vi "Storage Data.vi"(8 "Error In":errorcluster, 9 "Time Out In ms":i32=-1, 10 "Data In":variant, 11 "1D U16 Group With ID DVR Queue in":refnum<class "2D U16 Group With ID DVR Queue.lvclass">) -> (0 "Error Out":errorcluster, 1 "Time Out":bool, 3 "1D U16 Group With ID DVR Queue out":refnum<class "2D U16 Group With ID DVR Queue.lvclass">)   [LabVIEW 2024, in "2D U16 Group With ID DVR Queue.lvclass"]
uses:
  2D U16 Group With ID DVR Queue.lvclass
  Type Def/Data Type.ctl
  2D U16 Group With ID DVR Queue.lvclass/2D U16 Group With ID DVR Queue.ctl
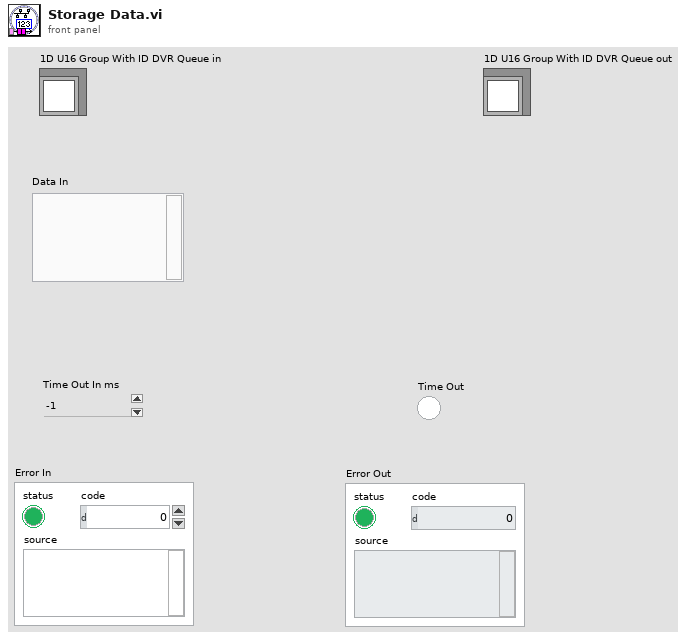
[diagram p1: front panel]
types:
  T1 = typedef "Data Type.ctl" = cluster{"Data ID":i64, "U16 Data Group":cluster{"Array":u16[][]}[]}
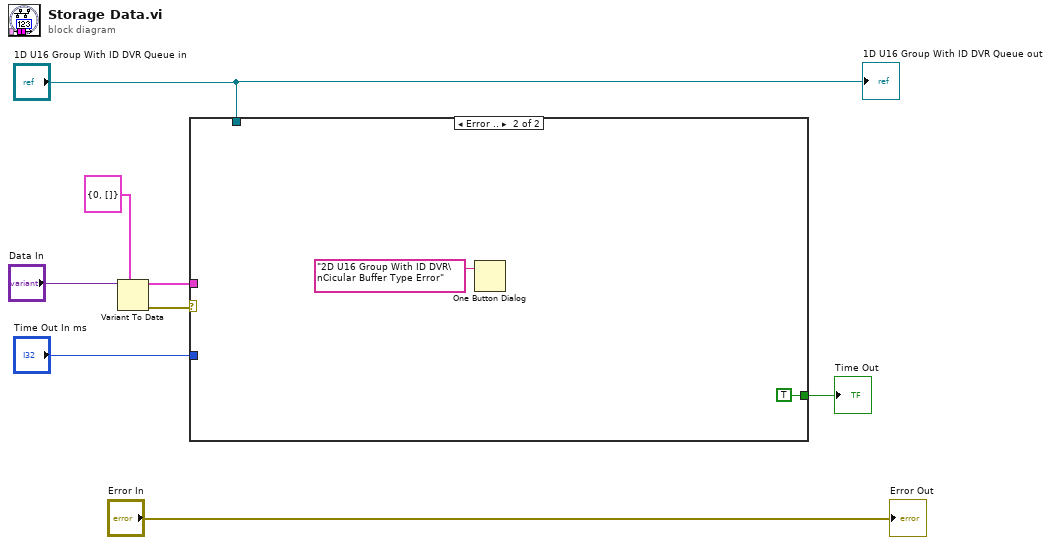
[diagram p0: block diagram]
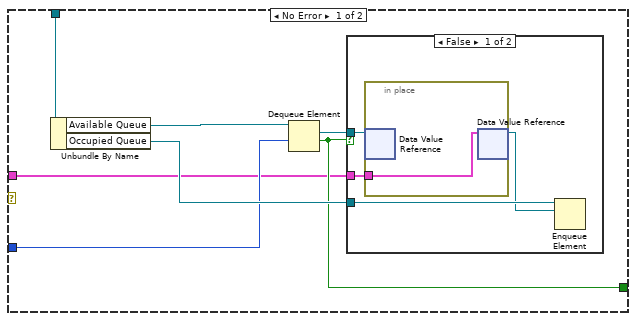
[diagram p2: hidden frame]
diagram:
  n1 = Variant To Data(type=T1 {"Data ID"=0, "U16 Data Group"=[]} ("Data In"), Variant="Data In") -> (data=w3:T1, error out=w1:errorcluster)  [unwired: 1 in]
  n2 = case shown="Error .." w1 {
    tunnel: "1D U16 Group With ID DVR Queue in" -> [w14 _]
    tunnel: [w11 TRUE ("timed out?")] -> w7
    tunnel: "Time Out In ms" -> [w10 _]
    tunnel: w3 -> [w9 _]
    frame No Error {
      n3 = Unbundle By Name(w14) -> ("Available Queue"=w13:refnum<queue>, "Occupied Queue"=w15:refnum<queue>)
      n4 = Dequeue Element(queue=w13, timeout in ms (-1)=w10) -> (element=w12:refnum<data-value>, timed out?=w11:bool)  [unwired: 1 in, 2 out]
      n5 = case shown="False" w11 {
        tunnel: w12 -> [w19 _]
        tunnel: w15 -> [w18 _]
        tunnel: w9 -> [w16 _]
        frame False {
          n6 = in-place {
            in-place-border: w16 -> [w20]
            n7 = in-place-dvr #1(w19) -> ()  [unwired: 2 out]
            n8 = in-place-dvr #1(w20) -> (w17:refnum<data-value>)  [unwired: 1 out]
          }
          n9 = Enqueue Element(queue=w18, element=w17) -> ()  [unwired: 2 in, 3 out]
        }
        frame True {
        }
      }
    }
    frame Error {
      n10 = One Button Dialog(message="2D U16 Group With ID DVR\nCicular Buffer Type Error") -> ()  [unwired: 1 in, 1 out]
    }
  }
  "Time Out" <- w7
  "1D U16 Group With ID DVR Queue out" <- "1D U16 Group With ID DVR Queue in"
  "Error Out" <- "Error In"
